vi "AllowTDCHitsRead.vi"() -> ()   [LabVIEW 2016]
panel:
  out "AllowTDCHitsRead":bool
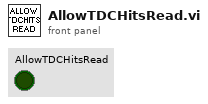
[diagram p1: front panel]
diagram:
